vi "HapticSPM_force_bonding_1D.vi"() -> ()   [LabVIEW 2023]
uses:
  Haptic-Programming-Interface/LabVIEW VIs/Haptic Prog Interface/Haptic Prog Interface.lvlib
panel:
  out "Stylus":refnum<vi>(3d-picture)
  out "Position":T1 {"z (mm)" format="%.1f"; "y (mm)" format="%.1f"; "x (mm)" format="%.1f"}
  out "3D Bonding Picture":refnum<vi>(3d-picture)
  out "k":dbl format="%#_13g"
  out "Setpoint":dbl format="%#_13g"
  out "Force Function":string
  in  "Input Function":i32 min=0 max=4 step=1
  out "Potential vs Distance":cluster{dbl[], dbl[]}(graph)
  out "Force vs Distance":cluster{dbl[], dbl[]}(graph)
  out "Z-Position (pm)":dbl caption="Numeric" min=0.0 format="%#.1p"
  out "Force":dbl(knob) scale=-4.0..4.0
  in  "Gain":dbl=1.0 caption="Numeric" format="%.1g"
  # "Super Ultra Mega Haptic SPM Controller 3000"
  # "Height"
  # "Move pen in all three dimensions to calibrate before feeling surface\n\nUse the \"PAGE UP\" or \"PAGE DOWN\" key to change the force function\n\nHold the pen as high as possible before changing force functions"
  # "Force"
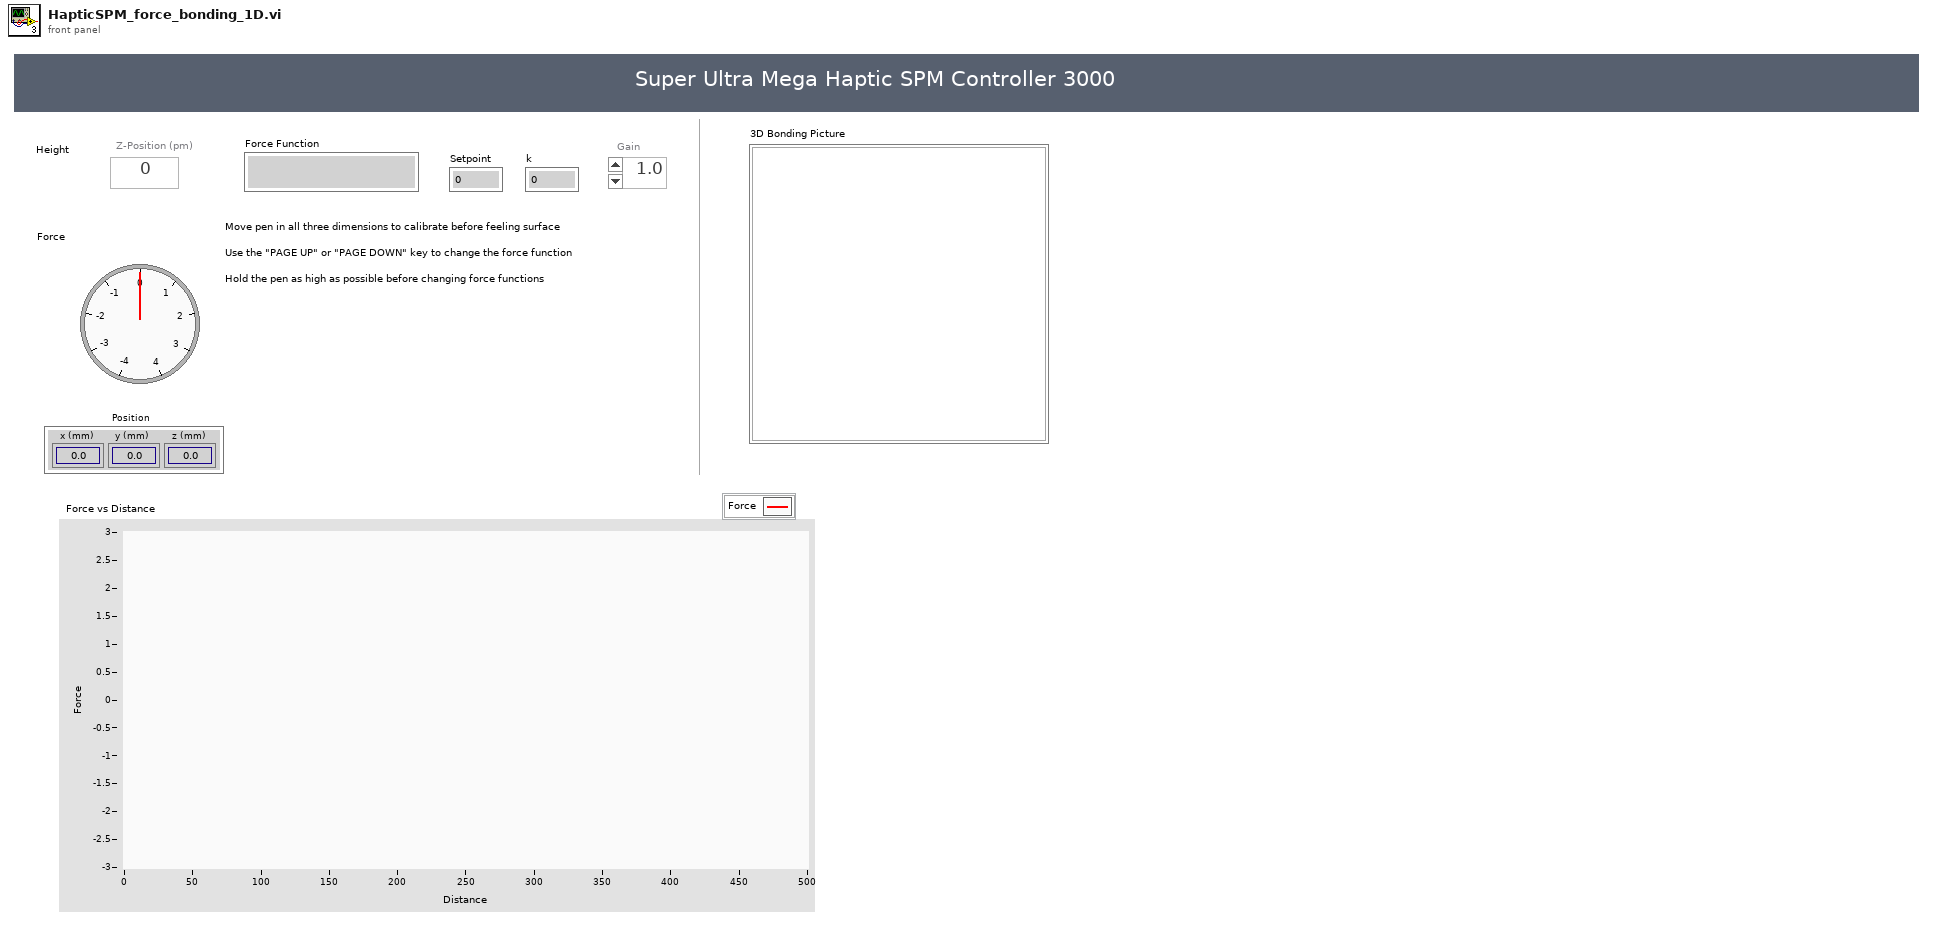
[diagram p1: front panel]
types:
  T1 = cluster{"x (mm)":dbl, "y (mm)":dbl, "z (mm)":dbl}
  T2 = cluster{"Fx (N)":dbl, "Fy (N)":dbl, "Fz (N)":dbl}
  T3 = cluster{"kx (N/m)":dbl, "ky (N/m)":dbl, "kz (N/m)":dbl}
  T4 = cluster{"X Drag":bool, "Y Drag":bool, "Z Drag":bool}
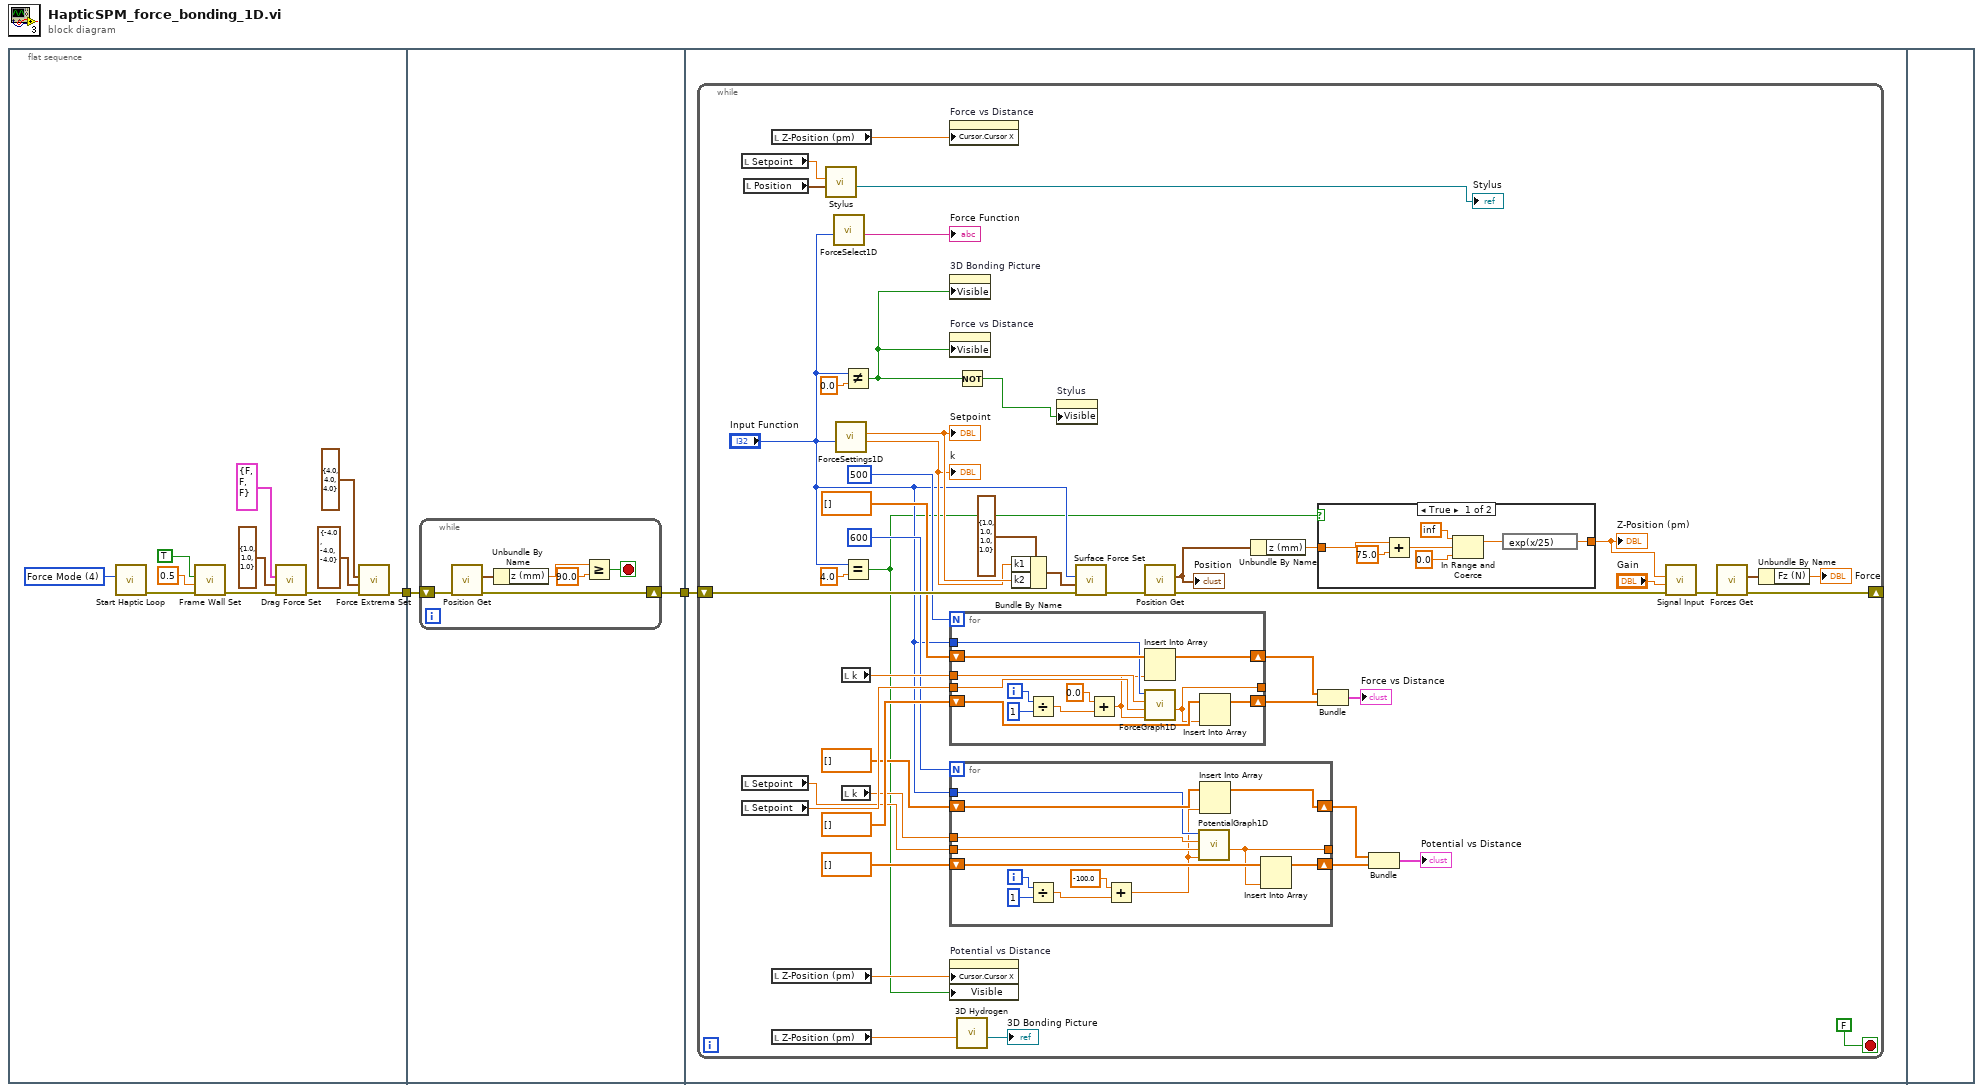
[diagram p0: block diagram]
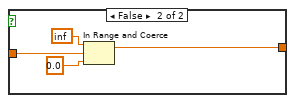
[diagram p2: hidden frame]
diagram:
  n1 = flat-sequence {
    tunnel: [w11] -> w2
    tunnel: w2 -> [w15]
    tunnel: [w14] -> w1
    tunnel: w1 -> [w22]
    frame #0 {
      w13 = u16 4 items=["Custom Mode", "Read Mode", "Write Mode", "Position Mode", "Force Mode"] ("Mode Selection")
      n2 = call "Start Haptic Loop.vi"("Mode Selection"=w13) -> ("error out"=w4:errorcluster)  [unwired: 10 in]
      n3 = call "Frame Wall Set.vi"("error in (no error)"=w4, "Wall Stiffness (N/m)"=0.5 ("Wall Stiffness"), "Restrict to Frame"=TRUE) -> ("error out"=w3:errorcluster)  [unwired: 8 in]
      n4 = call "Drag Force Set.vi"("error in (no error)"=w3, "Drag Coefficients (N/m)"=T3 {"kx (N/m)"=1.0, "ky (N/m)"=1.0, "kz (N/m)"=1.0} ("Drag Coefficients"), "Drag Force Toggles"=T4 {"X Drag"=FALSE, "Y Drag"=FALSE, "Z Drag"=FALSE}) -> ("error out"=w12:errorcluster)  [unwired: 8 in]
      n5 = call "Force Extrema Set.vi"("error in (no error)"=w12, "Minimum Force (N)"=T2 {"Fx (N)"=-4.0, "Fy (N)"=-4.0, "Fz (N)"=-4.0} ("Minimum Force"), "Maximum Force (N)"=T2 {"Fx (N)"=4.0, "Fy (N)"=4.0, "Fz (N)"=4.0} ("Maximum Force")) -> ("error out"=w11:errorcluster)  [unwired: 8 in]
    }
    frame #1 {
      n6 = while {
        shift-right: [w20] -> w14
        shift-left: w15 -> [w21]
        stop <- w16 stop-if-true
        n7 = call "Position Get.vi"("error in (no error)"=w21) -> ("error out"=w20:errorcluster, "Position"=w19:T1)  [unwired: 9 in]
        n8 = Unbundle By Name(w19) -> ("z (mm)"=w18:dbl)
        n9 = Greater Or Equal?(x=w18, y=90.0) -> (x >= y?=w16:bool)
      }
    }
    frame #2 {
      n10 = while {
        shift-right: [w52] -> _
        shift-left: w22 -> [w68]
        stop <- FALSE ("Boolean") stop-if-true
        n11 = local read "Setpoint"() -> (w29:dbl)
        n12 = local read "Setpoint"() -> (w43:dbl)
        n13 = local read "Setpoint"() -> (w54:dbl)
        n14 = local read "Position"() -> (w31:T1)
        n15 = local read "Z-Position (pm)"() -> (w53:dbl)
        n16 = local read "Z-Position (pm)"() -> (w42:dbl)
        n17 = local read "Z-Position (pm)"() -> (w35:dbl)
        n18 = call "Stylus.vi"("Position"=w31, "Radius"=w29) -> ("3D Picture"=→"Stylus":refnum<vi>)  [unwired: 8 in, 1 out]
        n19 = call "ForceSelect1D.vi"("Input Function"="Input Function") -> ("Force Function"=→"Force Function":string)  [unwired: 10 in]
        n20 = call "ForceSettings1D.vi"("Function"="Input Function") -> ("k"=w37:dbl, "Setpoint"=w38:dbl)  [unwired: 9 in]
        "Setpoint" <- w38
        "k" <- w37
        n21 = local read "k"() -> (w55:dbl)
        n22 = local read "k"() -> (w44:dbl)
        n23 = Not Equal?(x="Input Function", y=0.0) -> (x != y?=w28:bool)
        n24 = Equal?(x="Input Function", y=4.0) -> (x = y?=w25:bool)
        n25 = property on="Force vs Distance" class="XYGraph (strict)"("Cursor.Cursor X"=w53) -> ()  [unwired: 2 in, 2 out]
        n26 = property on="3D Bonding Picture" class="SceneGraphDisp (strict)"("Visible"=w28) -> ()  [unwired: 2 in, 2 out]
        n27 = property on="Force vs Distance" class="XYGraph (strict)"("Visible"=w28) -> ()  [unwired: 2 in, 2 out]
        n28 = for {
          N: 500 -> [_]
          shift-right: [w105] -> w60
          shift-left: dbl[] [] -> [w103]
          shift-right: [w104] -> w61
          shift-left: dbl[] [] -> [w102]
          tunnel: "Input Function" -> [w98]
          tunnel: [w101] -> _
          tunnel: w54 -> [w100]
          tunnel: w55 -> [w99]
          i -> [w96]
          n29 = Divide(x=w96, y=1) -> (x/y=w95:dbl)
          n30 = Add(x=0.0, y=w95) -> (x+y=w93:dbl)
          n31 = Insert Into Array(array=w102, new element=w93) -> (w104:dbl[])  [unwired: 1 in]
          n32 = call "ForceGraph1D.vi"("number"=w93, "Setpoint"=w100, "k"=w99, "Function"=w98) -> ("force"=w101:dbl)  [unwired: 7 in]
          n33 = Insert Into Array(array=w103, new element=w101) -> (w105:dbl[])  [unwired: 1 in]
        }
        n34 = for {
          N: 600 -> [_]
          shift-right: [w92] -> w49
          shift-left: dbl[] [] -> [w90]
          shift-right: [w91] -> w50
          shift-left: dbl[] [] -> [w89]
          tunnel: "Input Function" -> [w85]
          tunnel: [w88] -> _
          tunnel: w43 -> [w87]
          tunnel: w44 -> [w86]
          i -> [w83]
          n35 = Divide(x=w83, y=1) -> (x/y=w82:dbl)
          n36 = Add(x=-100.0, y=w82) -> (x+y=w80:dbl)
          n37 = call "PotentialGraph1D.vi"("number"=w80, "Setpoint"=w87, "k"=w86, "Function"=w85) -> ("potential"=w88:dbl)  [unwired: 7 in]
          n38 = Insert Into Array(array=w89, new element=w80) -> (w91:dbl[])  [unwired: 1 in]
          n39 = Insert Into Array(array=w90, new element=w88) -> (w92:dbl[])  [unwired: 1 in]
        }
        n40 = property on="Potential vs Distance" class="XYGraph (strict)"("Cursor.Cursor X"=w42, "Visible"=w25) -> ()  [unwired: 2 in, 2 out]
        n41 = Not(x=w28) -> (.not. x?=w23:bool)
        n42 = call "3D Hydrogen.vi"("Z-Position"=w35) -> ("reference out"=→"3D Bonding Picture":refnum<vi>)  [unwired: 10 in]
        n43 = Bundle By Name(cluster=cluster{"k1":dbl, "k2":dbl, "k3":dbl, "k4":dbl} {"k1"=1.0, "k2"=1.0, "k3"=1.0, "k4"=1.0} ("Force Constants"), "k1"=w37, "k2"=w38) -> (w64:cluster{"k1":dbl, "k2":dbl, "k3":dbl, "k4":dbl})
        n44 = property on="Stylus" class="SceneGraphDisp (strict)"("Visible"=w23) -> ()  [unwired: 2 in, 2 out]
        n45 = call "Surface Force Set.vi"("error in (no error)"=w68, "Force Constants"=w64, "Force Settings"="Input Function") -> ("error out"=w40:errorcluster)  [unwired: 8 in]
        n46 = call "Position Get.vi"("error in (no error)"=w40) -> ("error out"=w39:errorcluster, "Position"=w30:T1)  [unwired: 9 in]
        "Position" <- w30
        n47 = Unbundle By Name(w30) -> ("z (mm)"=w26:dbl)
        n48 = case shown="True" w25 {
          tunnel: [w69 w77] -> w27
          tunnel: w26 -> [w70 w76]
          frame True {
            n49 = Add(x=w70, y=75.0) -> (x+y=w74:dbl)
            n50 = In Range and Coerce(upper limit=inf, x=w74, lower limit=0.0) -> (coerced(x)=w75:dbl)  [unwired: 1 out]
            n51 = expression code="exp(x/25)"(w75) -> (w69:dbl)
          }
          frame False {
            n52 = In Range and Coerce(upper limit=inf, x=w76, lower limit=0.0) -> (coerced(x)=w77:dbl)  [unwired: 1 out]
          }
        }
        "Z-Position (pm)" <- w27
        n53 = Bundle(w61, w60) -> (→"Force vs Distance":cluster{dbl[], dbl[]})  [unwired: 1 in]
        n54 = Bundle(w50, w49) -> (→"Potential vs Distance":cluster{dbl[], dbl[]})  [unwired: 1 in]
        n55 = call "Signal Input.vi"("error in (no error)"=w39, "Gain"="Gain", "Signal"=w27) -> ("error out"=w67:errorcluster)  [unwired: 8 in]
        n56 = call "Forces Get.vi"("error in (no error)"=w67) -> ("error out"=w52:errorcluster, "Force (N)"=w63:T2)  [unwired: 9 in]
        n57 = Unbundle By Name(w63) -> ("Fz (N)"=→"Force":dbl)
      }
    }
    frame #3 {
    }
  }
